vi "[GV]_LIDAR Ethernet Address.vi"() -> ()   [LabVIEW 2016]
panel:
  in  "Lidar address":string="192.168.0.204"
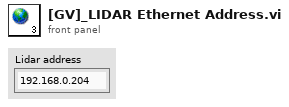
[diagram p1: front panel]
diagram:
